vi "R2100_Controller.vi"() -> ()   [LabVIEW 2016]
doc: "Controlls the R2100 LIDAR. Waits for a run signal from the ROS subscriber then initializes the UART before entering a loop where it reads the distance data on the lidar until a message to stop is received from the ROS subscriber."
uses:
  <vilib>/myRIO/Instrument Drivers/Onboard IO/DIO/typedefs/DIO Reference.ctl
  <vilib>/myRIO/Common/Instrument Driver Framework/Utilities/typedefs/myRIO Generic Hardware Reference.ctl
  <vilib>/myRIO/Common/Instrument Driver Framework/Utilities/typedefs/Hardware Version Enum.ctl
  <vilib>/myRIO/Common/Instrument Driver Framework/Utilities/typedefs/myRIO v1.0 Reference.ctl
  <vilib>/myRIO/Common/Instrument Driver Framework/Utilities/typedefs/Generic FPGA Reference.ctl
  <vilib>/myRIO/Common/Instrument Driver Framework/myRIO v1.0/DIO/typedefs/DIO Channels List.ctl
  <vilib>/myRIO/Common/Instrument Driver Framework/myRIO v1.0/DIO/typedefs/DIO Channels Enum.ctl
  <vilib>/userdefined/High Color/nirio_resource_hc.ctl
  <vilib>/myRIO/Instrument Drivers/Onboard IO/UART/typedef/VISA Configuration.ctl
  <vilib>/myRIO/Common/Instrument Driver Framework/Utilities/vis/Is FPGA Ref Available.vi
  <vilib>/myRIO/Common/Instrument Driver Framework/roboRIO v1.0/DIO/vis/roboRIO v1.0 Open DIO.vi
  <vilib>/myRIO/Instrument Drivers/Onboard IO/DIO/vis/Write.vi
  <vilib>/myRIO/Common/Instrument Driver Framework/Utilities/vis/Validate Channels.vi
  <vilib>/myRIO/Common/Instrument Driver Framework/roboRIO v1.0/DIO/vis/roboRIO v1.0 Reserve DIO.vi
  <vilib>/myRIO/Common/Instrument Driver Framework/roboRIO v1.0/DIO/vis/roboRIO v1.0 Build MUX Configuration DIO.vi
  <vilib>/myRIO/Common/Instrument Driver Framework/roboRIO v1.0/Resource Manager/vis/roboRIO v1.0 Reserve Channel List.vi
  <vilib>/myRIO/Common/Instrument Driver Framework/roboRIO v1.0/Resource Manager/vis/roboRIO v1.0 Create Configuration List.vi
  <vilib>/myRIO/Common/Instrument Driver Framework/roboRIO v1.0/Resource Manager/vis/roboRIO v1.0 Reserve Channel.vi
  <vilib>/myRIO/Common/Instrument Driver Framework/roboRIO v1.0/Resource Manager/vis/roboRIO v1.0 Unreserve Channel.vi
  <vilib>/myRIO/Common/Instrument Driver Framework/roboRIO v1.0/Resource Manager/vis/roboRIO v1.0 Build Mutex Name.vi
  GlobalVI.vi
  <vilib>/Utility/VariantDataType/GetNumericInfo.vi
  <vilib>/Utility/error.llb/Error Cluster From Error Code.vi
  <vilib>/myRIO/Common/Instrument Driver Framework/roboRIO v1.0/roboRIO v1.0 Open.vi
  <vilib>/myRIO/Common/Instrument Driver Framework/Utilities/vis/IO Manager.vi
  <vilib>/myRIO/Common/Instrument Driver Framework/Utilities/vis/Configuration Manager.vi
  <vilib>/myRIO/Common/Instrument Driver Framework/roboRIO v1.0/Resource Manager/vis/roboRIO v1.0 Configure IO.vi
  <vilib>/myRIO/Common/Instrument Driver Framework/myRIO v1.0/myRIO v1.0 Close.vi
  <vilib>/myRIO/Common/Instrument Driver Framework/roboRIO v1.0/DIO/vis/roboRIO v1.0 Write DIO.vi
  <vilib>/Instr/_visa.llb/VISA Configure Serial Port (Instr).vi
  <vilib>/myRIO/Express VI/Onboard Devices/LED/LED Express VI.xnode
  <vilib>/myRIO/Instrument Drivers/Onboard IO/DIO/vis/myRIO DIO Open.xnode
  <vilib>/myRIO/Instrument Drivers/Onboard IO/UART/UART.lvlib
  <vilib>/myRIO/Instrument Drivers/Onboard IO/DIO/DIO.lvlib
panel:
  out "range 11":u16(slide)
  out "range 10":u16(slide)
  out "range 9":u16(slide)
  out "range 8":u16(slide)
  out "range 7":u16(slide)
  out "range 6":u16(slide)
  out "range 5":u16(slide)
  out "range 4":u16(slide)
  out "range 3":u16(slide)
  out "range 2":u16(slide)
  out "noMsgs":bool
  out "syncCorrection":bool
  out "syncError":bool
  out "timeoutError":bool
  out "start_count":dbl
  out "timeout_count":dbl
  out "range":u16(slide)
  in  "Force Start":bool
  out "ROS Err Out":errorcluster
  out "AVG Range":dbl
  out "Distance_10":u16
  out "Distance_9":u16
  out "Distance_8":u16
  out "Distance_7":u16
  out "Distance_6":u16
  out "Distance_5":u16
  out "Distance_4":u16
  out "Distance_3":u16
  out "Distance_2":u16
  out "Distance_1":u16
  out "Distance_0":u16
  out "Msg Length":i32
  out "Output byte array":u8[](array[numeric]) format="%x"
  out "OUTPUT Err out":errorcluster
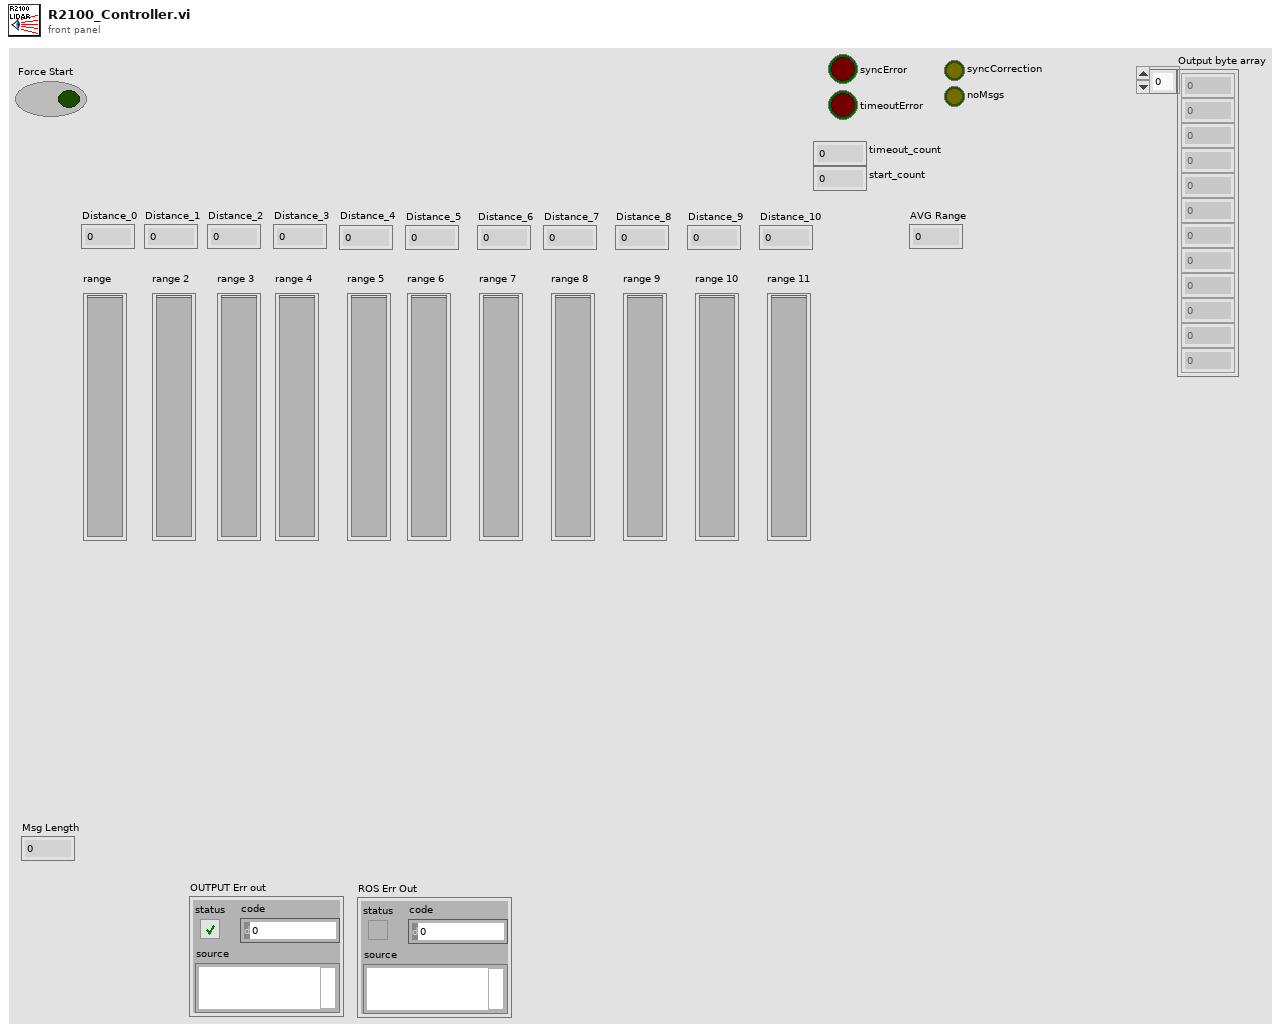
[diagram p1: front panel]
types:
  T1 = typedef "DIO.lvlib/DIO Reference.ctl" = cluster{"myRIO Reference":T2, "DIO Channels List":T6}
  T2 = typedef "myRIO Generic Hardware Reference.ctl" = cluster{"myRIO Model":T3, "myRIO Hardware Reference":T4}
  T3 = typedef "Hardware Version Enum.ctl" = enum16{"Unknown", "myRIO-1900", "myRIO-1950", "roboRIO", "NI ELVIS RIO CM"}
  T4 = typedef "myRIO v1.0 Reference.ctl" = cluster{"Generic FPGA Reference":T5, "Allow multiple opens":bool}
  T5 = typedef "Generic FPGA Reference.ctl" = refnum<k20>
  T6 = typedef "DIO Channels List.ctl" = T7[]
  T7 = typedef "DIO Channels Enum.ctl" = enum16{"Not Connected", "C/DIO0", "C/DIO1", "C/DIO2", "C/DIO3", "C/DIO4", "C/DIO5", "C/DIO6", "C/DIO7", "A/DIO0", "A/DIO1", "A/DIO2", "A/DIO3", "A/DIO4", "A/DIO5", "A/DIO6", "A/DIO7", "A/DIO8", "A/DIO9", "A/DIO10", "A/DIO11", "A/DIO12", "A/DIO13", "A/DIO14", "A/DIO15", "B/DIO0", "B/DIO1", "B/DIO2", "B/DIO3", "B/DIO4", "B/DIO5", "B/DIO6", "B/DIO7", "B/DIO8", "B/DIO9", "B/DIO10", "B/DIO11", "B/DIO12", "B/DIO13", "B/DIO14", "B/DIO15", "LED0", "LED1", "LED2", "LED3", "Button0", "DIO/DIO0", "DIO/DIO1", "DIO/DIO2", "DIO/DIO3", "DIO/DIO4", "DIO/DIO5", "DIO/DIO6", "DIO/DIO7", "DIO/DIO8", "DIO/DIO9", "SPI/CS0", "SPI/CS1", "SPI/CS2", "SPI/CS3", "LED RADIO (Green)", "LED RADIO (Red)", "LED COMM (Green)", "LED COMM (Red)", "LED MODE (Green)", "LED MODE (Red)"}
  T8 = typedef "nirio_resource_hc.ctl" = tag
  T9 = typedef "UART.lvlib/VISA Configuration.ctl" = cluster{"baud rate (9600)":u32, "data bits (8)":u16, "parity (0:none)":enum16{"None", "Odd", "Even", "Mark", "Space"}, "stop bits (10: 1 bit)":u16, "flow control (0:none)":u16, "termination char\n(0xA = '\\n' = LF) ":u8, "Enable Termination\nChar (T)":bool, "timeout (10sec)":u32}
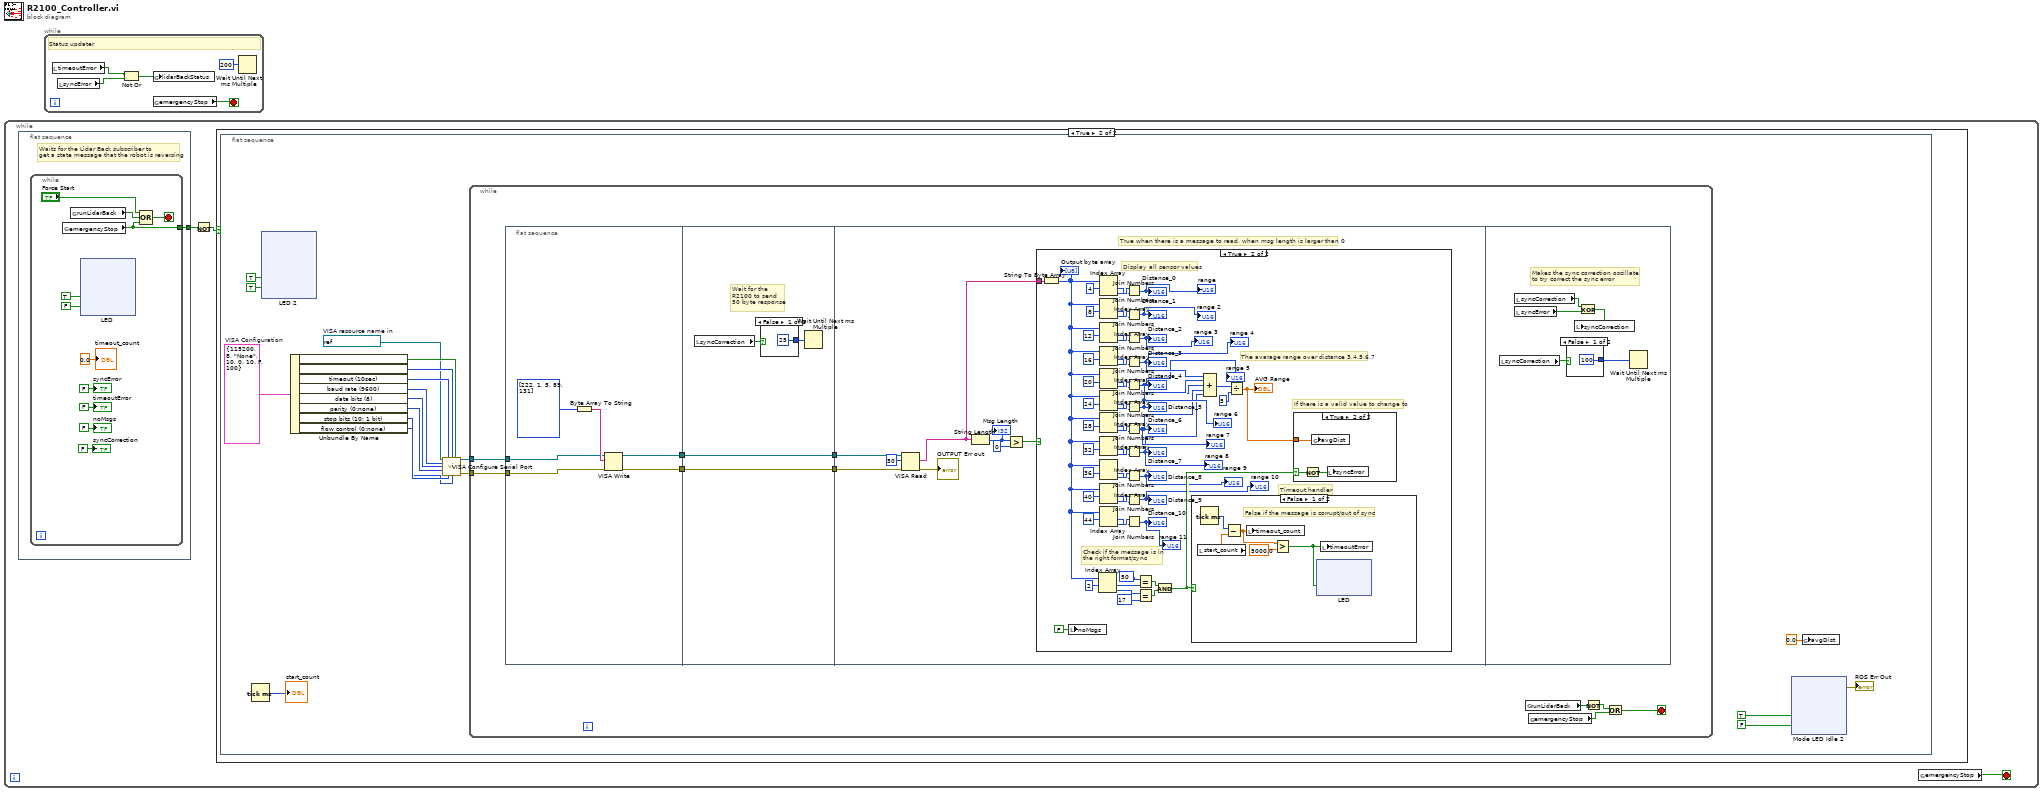
[diagram p0: block diagram]
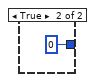
[diagram p3: hidden frame]
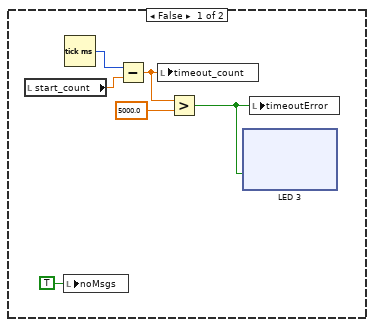
[diagram p4: hidden frame]
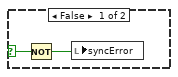
[diagram p5: hidden frame]
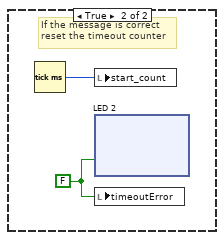
[diagram p6: hidden frame]
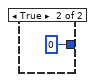
[diagram p7: hidden frame]
diagram:
  n1 = while {
    stop <- w3 stop-if-true
    n2 = flat-sequence {
      tunnel: [w313] -> w2
      frame #0 {
        # "Waits for the Lidar Back subscriber to\nget a state message that the robot is reversing"
        n3 = while {
          tunnel: [w320] -> w313
          stop <- w318 stop-if-true
          n4 = global read "GlobalVI.vi" "emergencyStop"() -> (w320:bool)
          n5 = global read "GlobalVI.vi" "runLidarBack"() -> (w321:bool)
          n6 = xnode "LED"("ModeG"=TRUE ("Mode"), "ModeR"=FALSE) -> ()  [unwired: 1 in, 1 out]
          n7 = Compound Arithmetic op=OR("Force Start", w321, w320) -> (w318:bool)
          "timeout_count" <- 0.0 ("Timeout_count")
          "syncError" <- FALSE ("syncError")
          "timeoutError" <- FALSE ("timeoutError")
          "noMsgs" <- FALSE ("noMsgs")
          "syncCorrection" <- FALSE ("syncCorrection")
        }
      }
    }
    n8 = Not(x=w2) -> (.not. x?=w1:bool)
    n9 = case shown="True" w1 {
      frame False {
      }
      frame True {
        n10 = flat-sequence {
          frame #0 {
            w8 = T9 {"baud rate (9600)"=115200, "data bits (8)"=8, "parity (0:none)"=enum."None", "stop bits (10: 1 bit)"=10, "flow control (0:none)"=0, "termination char\n(0xA = '\\n' = LF) "=10, "Enable Termination\nChar (T)"=FALSE, "timeout (10sec)"=100}  # VISA Configuration
            w7 = refnum<visa-resource-name> "ASRL1::INSTR"  # VISA resource name in
            n11 = Tick Count (ms)() -> (millisecond timer value=→"start_count":u32)
            n12 = xnode "LED 2"("ModeG"=TRUE ("Mode"), "ModeR"=TRUE) -> ()  [unwired: 1 in, 1 out]
            n13 = Unbundle By Name(w8) -> ("Enable Termination\nChar (T)"=w9:bool, "termination char\n(0xA = '\\n' = LF)"=w10:u8, "timeout (10sec)"=w11:u32, "baud rate (9600)"=w16:u32, "data bits (8)"=w15:u16, "parity (0:none)"=w14:enum16{"None", "Odd", "Even", "Mark", "Space"}, "stop bits (10: 1 bit)"=w13:u16, "flow control (0:none)"=w12:u16)
            n14 = call-poly "VISA Configure Serial Port"("VISA resource name"=w7, "timeout (10sec)"=w11, "termination char\n(0xA = '\\n' = LF)"=w10, "Enable Termination\nChar (T)"=w9, "baud rate (9600)"=w16, "data bits (8)"=w15, "parity (0:none)"=w14, "stop bits (10: 1 bit)"=w13, "flow control (0:none)"=w12) -> ("VISA resource name out"=w6:refnum<visa-resource-name>, "error out"=w5:errorcluster)  [unwired: 5 in]
            n15 = while {
              tunnel: w6 -> [w100]
              tunnel: w5 -> [w99]
              stop <- w104 stop-if-true
              n16 = flat-sequence {
                tunnel: w100 -> [w108]
                tunnel: w99 -> [w107]
                tunnel: [w106] -> w97
                tunnel: [w105] -> w95
                tunnel: [w112] -> w98
                tunnel: w97 -> [w112]
                tunnel: [w111] -> w96
                tunnel: w95 -> [w111]
                tunnel: w98 -> [w118]
                tunnel: w96 -> [w117]
                frame #0 {
                  n17 = Byte Array To String(unsigned byte array=u8[] [222, 1, 5, 89, 131]) -> (string=w109:string)
                  n18 = VISA Write(VISA resource name=w108, write buffer=w109, error in (no error)=w107) -> (VISA resource name out=w106:refnum<visa-resource-name>, error out=w105:errorcluster)  [unwired: 1 out]
                }
                frame #1 {
                  # "Wait for the \nR2100 to send\n50 byte response"
                  n19 = local read "syncCorrection"() -> (w114:bool)
                  n20 = case shown="False" w114 {
                    tunnel: [u32 25 ("milliseconds to wait") u32 0 ("milliseconds to wait")] -> w113
                    frame False {
                    }
                    frame True {
                    }
                  }
                  n21 = Wait Until Next ms Multiple(millisecond multiple=w113) -> ()  [unwired: 1 out]
                }
                frame #2 {
                  # "True when there is a message to read, when msg length is larger than 0"
                  n22 = VISA Read(VISA resource name=w118, byte count=u32 50, error in (no error)=w117) -> (read buffer=w124:string, error out=→"OUTPUT Err out":errorcluster)  [unwired: 2 out]
                  n23 = String Length(string=w124) -> (length=w121:i32)
                  "Msg Length" <- w121
                  n24 = Greater?(x=w121, y=0) -> (0:w119:bool)
                  n25 = case shown="True" w119 {
                    tunnel: w124 -> [_ w223]
                    frame False {
                      n26 = local read "start_count"() -> (w129:dbl)
                      n27 = local write "noMsgs"(TRUE ("noMsgs")) -> ()
                      n28 = Tick Count (ms)() -> (millisecond timer value=w130:u32)
                      n29 = Subtract(x=w130, y=w129) -> (x-y=w126:dbl)
                      n30 = local write "timeout_count"(w126) -> ()
                      n31 = Greater?(x=w126, y=5000.0) -> (0:w127:bool)
                      n32 = xnode "LED 3"("RADIO (Red)"=w127) -> ()  [unwired: 1 in, 1 out]
                      n33 = local write "timeoutError"(w127) -> ()
                    }
                    frame True {
                      # "If there is a valid value to change to"
                      # "Timeout handler"
                      # "Check if the message is in\nthe right format/sync"
                      # "Display all sensor values"
                      # "The avarage range over distance 3,4,5,6,7"
                      n34 = String To Byte Array(string=w223) -> (unsigned byte array=w186:u8[])
                      "Output byte array" <- w186
                      n35 = local write "noMsgs"(FALSE ("noMsgs")) -> ()
                      n36 = Index Array(array=w186, index #1=2 ("index")) -> (element #1=w185:u8, element #2=w184:u8)  [unwired: 1 in]
                      n37 = Index Array(array=w186, index #1=4 ("index")) -> (element #1=w220:u8, element #2=w221:u8)  [unwired: 1 in]
                      n38 = Index Array(array=w186, index #1=8 ("index")) -> (element #1=w217:u8, element #2=w218:u8)  [unwired: 1 in]
                      n39 = Index Array(array=w186, index #1=12 ("index")) -> (element #1=w214:u8, element #2=w215:u8)  [unwired: 1 in]
                      n40 = Index Array(array=w186, index #1=16 ("index")) -> (element #1=w211:u8, element #2=w212:u8)  [unwired: 1 in]
                      n41 = Index Array(array=w186, index #1=20 ("index")) -> (element #1=w208:u8, element #2=w209:u8)  [unwired: 1 in]
                      n42 = Index Array(array=w186, index #1=24 ("index")) -> (element #1=w205:u8, element #2=w206:u8)  [unwired: 1 in]
                      n43 = Index Array(array=w186, index #1=28 ("index")) -> (element #1=w202:u8, element #2=w203:u8)  [unwired: 1 in]
                      n44 = Index Array(array=w186, index #1=32 ("index")) -> (element #1=w199:u8, element #2=w200:u8)  [unwired: 1 in]
                      n45 = Index Array(array=w186, index #1=36 ("index")) -> (element #1=w196:u8, element #2=w197:u8)  [unwired: 1 in]
                      n46 = Index Array(array=w186, index #1=40 ("index")) -> (element #1=w193:u8, element #2=w194:u8)  [unwired: 1 in]
                      n47 = Index Array(array=w186, index #1=44 ("index")) -> (element #1=w190:u8, element #2=w191:u8)  [unwired: 1 in]
                      n48 = Join Numbers(hi=w221, lo=w220) -> ((hi.lo)=→"Distance_0" →"range":u16)
                      n49 = Join Numbers(hi=w218, lo=w217) -> ((hi.lo)=→"Distance_1" →"range 2":u16)
                      n50 = Join Numbers(hi=w215, lo=w214) -> ((hi.lo)=→"Distance_2" →"range 3":u16)
                      n51 = Join Numbers(hi=w212, lo=w211) -> ((hi.lo)=w174:u16)
                      "Distance_3" <- w174
                      "range 4" <- w174
                      n52 = Join Numbers(hi=w209, lo=w208) -> ((hi.lo)=w173:u16)
                      "Distance_4" <- w173
                      "range 5" <- w173
                      n53 = Join Numbers(hi=w206, lo=w205) -> ((hi.lo)=w172:u16)
                      "Distance_5" <- w172
                      "range 6" <- w172
                      n54 = Join Numbers(hi=w203, lo=w202) -> ((hi.lo)=w171:u16)
                      "Distance_6" <- w171
                      "range 7" <- w171
                      n55 = Join Numbers(hi=w200, lo=w199) -> ((hi.lo)=w170:u16)
                      "Distance_7" <- w170
                      "range 8" <- w170
                      n56 = Join Numbers(hi=w197, lo=w196) -> ((hi.lo)=→"Distance_8" →"range 9":u16)
                      n57 = Join Numbers(hi=w194, lo=w193) -> ((hi.lo)=→"Distance_9" →"range 10":u16)
                      n58 = Join Numbers(hi=w191, lo=w190) -> ((hi.lo)=→"Distance_10" →"range 11":u16)
                      n59 = Equal?(x=u8 50, y=w185) -> (x = y?=w181:bool)
                      n60 = Equal?(x=w184, y=u8 17) -> (x = y?=w180:bool)
                      n61 = And(x=w181, y=w180) -> (x .and. y?=w178:bool)
                      n62 = case shown="False" w178 {
                        frame False {
                          # "False if the message is corrupt/out of sync"
                          n63 = local read "start_count"() -> (w232:dbl)
                          n64 = Tick Count (ms)() -> (millisecond timer value=w233:u32)
                          n65 = Subtract(x=w233, y=w232) -> (x-y=w230:dbl)
                          n66 = local write "timeout_count"(w230) -> ()
                          n67 = Greater?(x=w230, y=5000.0 ("x")) -> (0:w229:bool)
                          n68 = xnode "LED"("RADIO (Red)"=w229) -> ()  [unwired: 1 in, 1 out]
                          n69 = local write "timeoutError"(w229) -> ()
                        }
                        frame True {
                          w269 = FALSE ("RADIO (Red)")
                          # "If the message is correct\nreset the timeout counter"
                          n70 = Tick Count (ms)() -> (millisecond timer value=w270:u32)
                          n71 = local write "start_count"(w270) -> ()
                          n72 = xnode "LED 2"("RADIO (Red)"=w269) -> ()  [unwired: 1 in, 1 out]
                          n73 = local write "timeoutError"(w269) -> ()
                        }
                      }
                      n74 = Compound Arithmetic op=ADD(w174, w173, w172, w171, w170) -> (w189:u16)
                      n75 = Divide(x=w189, y=u16 5) -> (x/y=w179:dbl)
                      "AVG Range" <- w179
                      n76 = case shown="True" w178 {
                        selector: w178 -> [w225 w228]
                        tunnel: w179 -> [_ w226]
                        frame False {
                          n77 = Not(x=w225) -> (.not. x?=w224:bool)
                          n78 = local write "syncError"(w224) -> ()
                        }
                        frame True {
                          n79 = Not(x=w228) -> (.not. x?=w227:bool)
                          n80 = global write "GlobalVI.vi" "avgDist"(w226) -> ()
                          n81 = local write "syncError"(w227) -> ()
                        }
                      }
                    }
                  }
                }
                frame #3 {
                  # "Makes the sync correction oscillate\nto try correct the sync error"
                  n82 = local read "syncCorrection"() -> (w306:bool)
                  n83 = local read "syncCorrection"() -> (w309:bool)
                  n84 = local read "syncError"() -> (w308:bool)
                  n85 = case shown="False" w306 {
                    tunnel: [u32 100 ("milliseconds to wait") u32 0 ("milliseconds to wait")] -> w310
                    frame False {
                    }
                    frame True {
                    }
                  }
                  n86 = Exclusive Or(1:w308, 2:w309) -> (0:w307:bool)
                  n87 = local write "syncCorrection"(w307) -> ()
                  n88 = Wait Until Next ms Multiple(millisecond multiple=w310) -> ()  [unwired: 1 out]
                }
              }
              n89 = global read "GlobalVI.vi" "runLidarBack"() -> (w102:bool)
              n90 = global read "GlobalVI.vi" "emergencyStop"() -> (w103:bool)
              n91 = Not(x=w102) -> (.not. x?=w101:bool)
              n92 = Or(x=w101, y=w103) -> (x .or. y?=w104:bool)
            }
            n93 = xnode "Mode LED Idle 2"("ModeG"=TRUE ("Mode"), "ModeR"=FALSE) -> ("error out"=→"ROS Err Out":errorcluster)  [unwired: 1 in]
            n94 = global write "GlobalVI.vi" "avgDist"(0.0 ("avgDist")) -> ()
          }
        }
      }
    }
    n95 = global read "GlobalVI.vi" "emergencyStop"() -> (w3:bool)
  }
  n96 = while {
    stop <- w365 stop-if-true
    # "Status updater"
    n97 = local read "timeoutError"() -> (w364:bool)
    n98 = local read "syncError"() -> (w363:bool)
    n99 = Not Or(1:w363, 2:w364) -> (0:w362:bool)
    n100 = global write "GlobalVI.vi" "lidarBackStatus"(w362) -> ()
    n101 = global read "GlobalVI.vi" "emergencyStop"() -> (w365:bool)
    n102 = Wait Until Next ms Multiple(millisecond multiple=u32 200) -> ()  [unwired: 1 out]
  }
